vi "GZip Decompress.vi"(8 "error in (no error)":errorcluster, 11 "GZip compressed string":string="Hello World!") -> (0 "error out":errorcluster, 3 "Decompressed string":string)   [LabVIEW 2015, in "LSR Transmission.lvlib"]
doc: "Returns the decompressed value of the GZip string input. Uses the Open G Zip Tools. Requires version 4.1.0-b2 or later for Linux RT support."
uses:
  LSR Transmission.lvlib
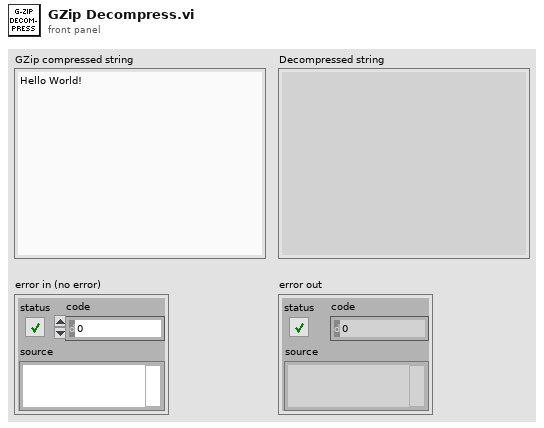
[diagram p1: front panel]
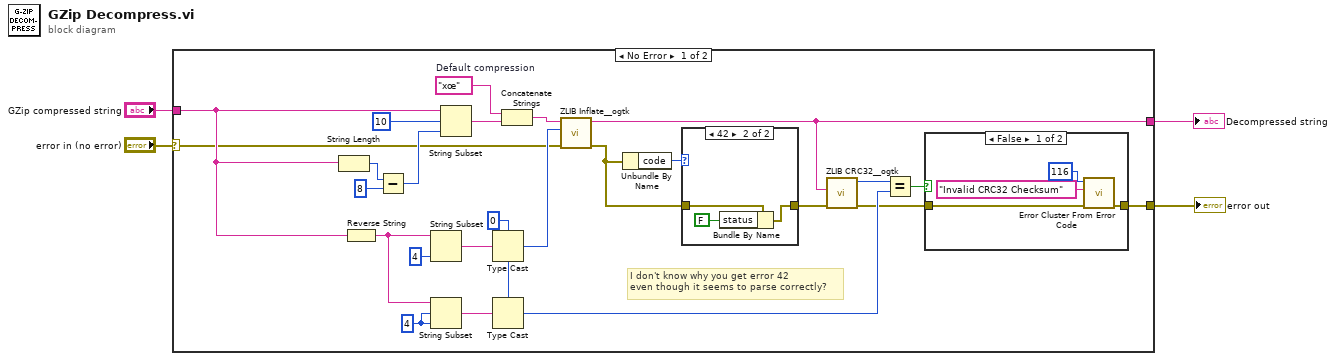
[diagram p0: block diagram]
diagram:
  n1 = case shown="No Error" "error in (no error)" {
    selector: "error in (no error)" -> [w8 w39]
    tunnel: "GZip compressed string" -> [w25 _]
    tunnel: [w18 _] -> w3
    tunnel: [w9 w39] -> w2
    frame No Error {
      w17 = "xœ"  # Default compression
      w19 = u32 0
      w22 = 4 ("length (rest)")
      # "I don't know why you get error 42\neven though it seems to parse correctly?"
      n2 = String Length(string=w25) -> (length=w28:i32)
      n3 = Reverse String(1:w25) -> (0:w23:string)
      n4 = Subtract(x=w28, y=8) -> (x-y=w26:i32)
      n5 = String Subset(string=w23, length (rest)=4 ("length (rest)")) -> (substring=w21:string)  [unwired: 1 in]
      n6 = String Subset(string=w23, offset (0)=w22, length (rest)=w22) -> (substring=w20:string)
      n7 = String Subset(string=w25, offset (0)=10, length (rest)=w26) -> (substring=w16:string)
      n8 = Type Cast(type=w19, x=w21) -> (*(type *) &x=w13:u32)
      n9 = Type Cast(type=w19, x=w20) -> (*(type *) &x=w12:u32)
      n10 = Concatenate Strings(w17, w16) -> (w15:string)
      n11 = call <userlib>:"ZLIB Inflate__ogtk.vi"("error in (no error)"=w8, "expected length (try out)"=w13, "input"=w15) -> ("error out"=w6:errorcluster, "inflated output"=w18:string)  [unwired: 2 in, 1 out]
      n12 = Unbundle By Name(w6) -> ("code"=w7:i32)
      n13 = case shown="42" w7 {
        tunnel: w6 -> [w30 w33]
        tunnel: [w30 w32] -> w5
        frame Default {
        }
        frame 42 {
          n14 = Bundle By Name(cluster=w33, "status"=FALSE) -> (w32:errorcluster)
        }
      }
      n15 = call <userlib>:"ZLIB CRC32__ogtk.vi"("error in (no error)"=w5, "buffer"=w18) -> ("error out"=w10:errorcluster, "new crc32"=w14:u32)  [unwired: 4 in]
      n16 = Equal?(x=w14, y=w12) -> (x = y?=w11:bool)
      n17 = case shown="False" w11 {
        tunnel: w10 -> [w36 w38]
        tunnel: [w37 w38] -> w9
        frame False {
          n18 = call <vilib>:"Error Cluster From Error Code.vi"("error in (no error)"=w36, "error message (\"\")"="Invalid CRC32 Checksum" ("error message (\"\")"), "error code (0)"=116) -> ("error out"=w37:errorcluster)  [unwired: 6 in]
        }
        frame True {
        }
      }
    }
    frame Error {
    }
  }
  "Decompressed string" <- w3
  "error out" <- w2
